vi "Wilkinson Matrix (DBL).vi"(11 "matrix size":i32) -> (0 "error":i32, 3 "Wilkinson Matrix":T1)   [LabVIEW 2020, in "NI_AALPro.lvlib"]
uses:
  NI_AALPro.lvlib
  RealMatrix.ctl
  NI_AALBase.lvlib
  NI_Matrix.lvlib
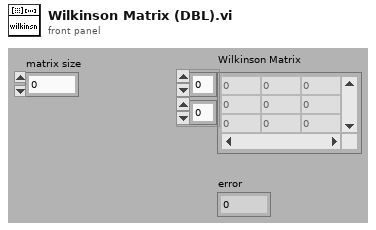
[diagram p1: front panel]
types:
  T1 = typedef "NI_Matrix.lvlib/RealMatrix.ctl" = dbl[][]
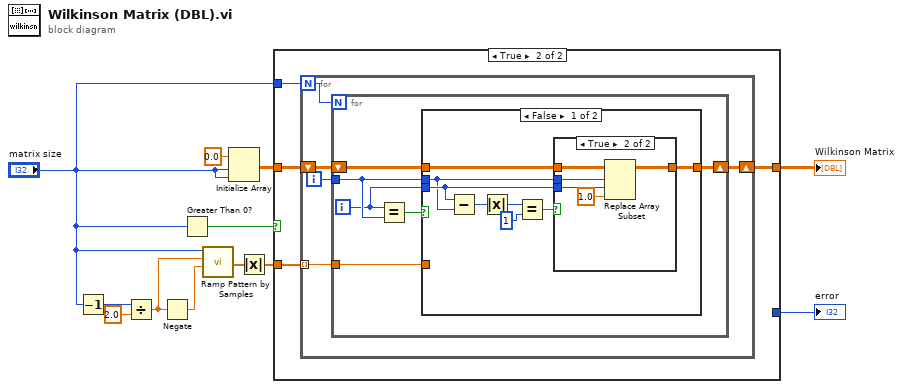
[diagram p0: block diagram]
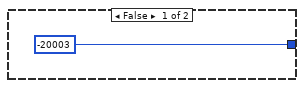
[diagram p2: hidden frame]
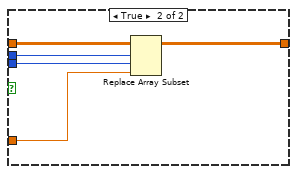
[diagram p4: hidden frame]
diagram:
  n1 = Decrement(x="matrix size") -> (x-1=w8:i32)
  n2 = Divide(x=w8, y=2.0) -> (x/y=w5:dbl)
  n3 = Negate(x=w5) -> (-x=w6:dbl)
  n4 = Greater Than 0?(x="matrix size") -> (x > 0?=w11:bool)
  n5 = call "Ramp Pattern by Samples.vi"("start"=w6, "end"=w5, "samples"="matrix size") -> ("Ramp Pattern"=w4:dbl[])  [unwired: 7 in, 1 out]
  n6 = Initialize Array(0.0 ("element"), "matrix size", "matrix size") -> (w9:dbl[][])
  n7 = Absolute Value(x=w4) -> (abs(x)=w3:dbl[])
  n8 = case shown="True" w11 {
    tunnel: [_ w17] -> w1
    tunnel: [-20003 _] -> w12
    tunnel: w9 -> [_ w16]
    tunnel: "matrix size" -> [_ w15]
    tunnel: w3 -> [_ w14]
    frame False {
    }
    frame True {
      n9 = for {
        N: w15 -> [w18]
        shift-right: [w20] -> w17
        shift-left: w16 -> [w21]
        tunnel: w14 -> [w19] mode=indexing
        i -> [w22]
        n10 = for {
          N: w18 -> [_]
          tunnel: w22 -> [w25]
          shift-right: [w23] -> w20
          shift-left: w21 -> [w26]
          tunnel: w19 -> [w27]
          i -> [w24]
          n11 = Equal?(x=w24, y=w25) -> (x = y?=w28:bool)
          n12 = case shown="False" w28 {
            tunnel: [w31 w47] -> w23
            tunnel: w26 -> [w32 w46]
            tunnel: w27 -> [_ w45]
            tunnel: w25 -> [w29 w44]
            tunnel: w24 -> [w30 w43]
            frame False {
              n13 = Subtract(x=w30, y=w29) -> (x-y=w36:i32)
              n14 = Absolute Value(x=w36) -> (abs(x)=w35:i32)
              n15 = Equal?(x=w35, y=1) -> (x = y?=w33:bool)
              n16 = case shown="True" w33 {
                tunnel: w32 -> [w37 w38]
                tunnel: [w37 w39] -> w31
                tunnel: w30 -> [_ w41]
                tunnel: w29 -> [_ w42]
                frame False {
                }
                frame True {
                  n17 = Replace Array Subset(array=w38, new element=1.0, index (row)=w42, index (col)=w41) -> (w39:dbl[][])
                }
              }
            }
            frame True {
              n18 = Replace Array Subset(array=w46, new element=w45, index (row)=w44, index (col)=w43) -> (w47:dbl[][])
            }
          }
        }
      }
    }
  }
  "error" <- w12
  "Wilkinson Matrix" <- w1
